vi "MockFAILC4.vi"(11 "MockFAILC4Settings":T1={"ModbusTxDataFIFO"="ModbusSubnetDTxDataFIFO", "Code17Memory"="MockFAILC4Code17", "BufferUpdateFIFO"="MockFAILC4Command", "ModbusRxDataFIFO"="ModbusSubnetDRxDataFIFO", "Code18Memory"="MockFAILC4Code18", "Code65Memory"="MockFAILC4Code65", "Code66Memory"="MockFAILC4Code66", "Code67Memory"="MockFAILC4Code67", "Code72Memory"="MockFAILC4Code72", "Code80Memory"="MockFAILC4Code80", "Code110Memory"="MockFAILC4Code110", "CRCDataFIFO"="MockFAILC4CRCDataFIFO", "CRCCalculateFIFO"="MockFAILC4CRCCalculateFIFO", "CRCFIFO"="MockFAILC4CRCFIFO"}) -> ()   [LabVIEW 2018, in "FPGAMockFAILC.lvlib"]
uses:
  FPGAMockFAILC.lvlib
  Common_FPGA_Modbus/DataTypes/ModbusCRCSettings.ctl
  DataTypes/MockFAILC4Settings.ctl
  Common_FPGA_Modbus/FPGAModbus.lvlib
panel:
  in  "ModbusCRCSettings":T2={"DataFIFO"="MockFAILC4CRCDataFIFO", "CalculateFIFO"="MockFAILC4CRCCalculateFIFO", "OutputFIFO"="MockFAILC4CRCFIFO"}
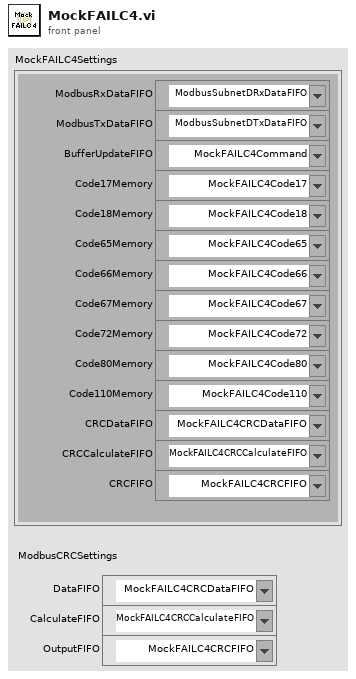
[diagram p1: front panel]
types:
  T1 = typedef "FPGAMockFAILC.lvlib/MockFAILC4Settings.ctl" = cluster{"ModbusTxDataFIFO":refnum<k21>, "Code17Memory":refnum<k21>, "BufferUpdateFIFO":refnum<k21>, "ModbusRxDataFIFO":refnum<k21>, "Code18Memory":refnum<k21>, "Code65Memory":refnum<k21>, "Code66Memory":refnum<k21>, "Code67Memory":refnum<k21>, "Code72Memory":refnum<k21>, "Code80Memory":refnum<k21>, "Code110Memory":refnum<k21>, "CRCDataFIFO":refnum<k21>, "CRCCalculateFIFO":refnum<k21>, "CRCFIFO":refnum<k21>}
  T2 = typedef "FPGAModbus.lvlib/ModbusCRCSettings.ctl" = cluster{"DataFIFO":refnum<k21>, "CalculateFIFO":refnum<k21>, "OutputFIFO":refnum<k21>}
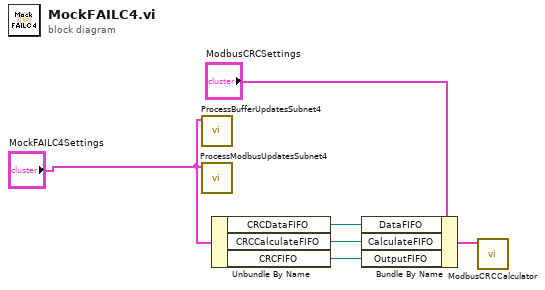
[diagram p0: block diagram]
diagram:
  n1 = call "ProcessBufferUpdatesSubnet4.vi"("MockFAILC4Settings"="MockFAILC4Settings") -> ()  [unwired: 11 in]
  n2 = call "ProcessModbusUpdatesSubnet4.vi"("MockFAILC4Settings"="MockFAILC4Settings") -> ()  [unwired: 11 in]
  n3 = Unbundle By Name("MockFAILC4Settings") -> ("CRCDataFIFO"=w3:refnum<k21>, "CRCCalculateFIFO"=w4:refnum<k21>, "CRCFIFO"=w5:refnum<k21>)
  n4 = Bundle By Name(cluster="ModbusCRCSettings", "DataFIFO"=w3, "CalculateFIFO"=w4, "OutputFIFO"=w5) -> (w6:T2)
  n5 = call "ModbusCRCCalculator.vi"("ModbusCRCSettings"=w6) -> ()  [unwired: 11 in]
